vi "DPO_7K_Set_Channel_Bandwidth.vi"(8 "Error In":errorcluster, 9 "Bandwidth":u16(ring) items=["500 MHz", "1 GHz", "2 GHz", "3 GHz", "4 GHz", "5 GHz", "6 GHz", "7 GHz", "8 GHz", "9 GHz", "10 GHz", "11 GHz", "12 GHz", "13 GHz", "14 GHz", "15 GHz", "16 GHz", "17 GHz", "18 GHz", "19 GHz", "20 GHz", "21 GHz", "22 GHz", "23 GHz", "24 GHz", "25 GHz", "26 GHz", "27 GHz", "28 GHz", "29 GHz", "30 GHz", "31 GHz", "32 GHz", "33 GHz", "33 GHz HW (Tek)", "34 GHz (ATI)", "35 GHz (ATI)", "36 GHz (ATI)", "38 GHz (ATI)", "40 GHz (ATI)", "45 GHz (ATI)", "50 GHz (ATI)"], 10 "Channel":u16(ring) items=["Channel 1", "Channel 2", "Channel 3", "Channel 4", "Math 1", "Math 2", "Math 3", "Math 4", "Reference 1", "Reference 2", "Reference 3", "Reference 4"], 11 "VISA resource name in":refnum<visa-resource-name>) -> (0 "Error Out":errorcluster, 3 "VISA resource name out":refnum<visa-resource-name>)   [LabVIEW 2020]
uses:
  subVI/Return_To_Interface.ctl
  subVI/Set_Configuration.ctl
panel:
  in  "Set":T1
  in  "Return to Interface":T2
  # "SET CHANNEL BANDWIDTH"
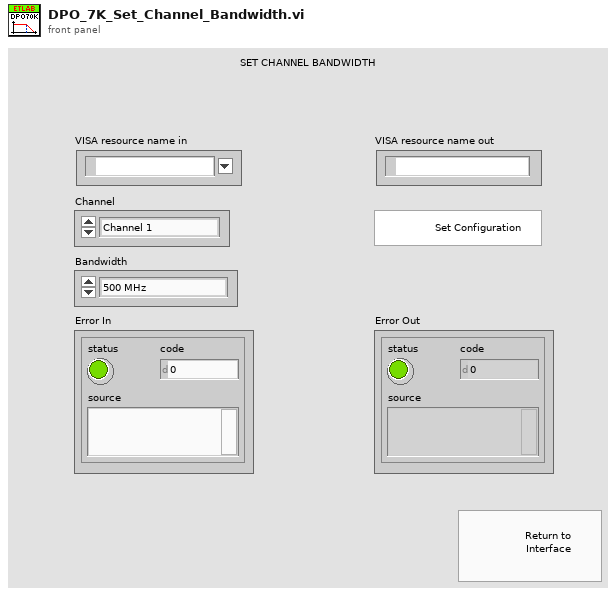
[diagram p1: front panel]
types:
  T1 = typedef "Set_Configuration.ctl" = bool
  T2 = typedef "Return_To_Interface.ctl" = bool
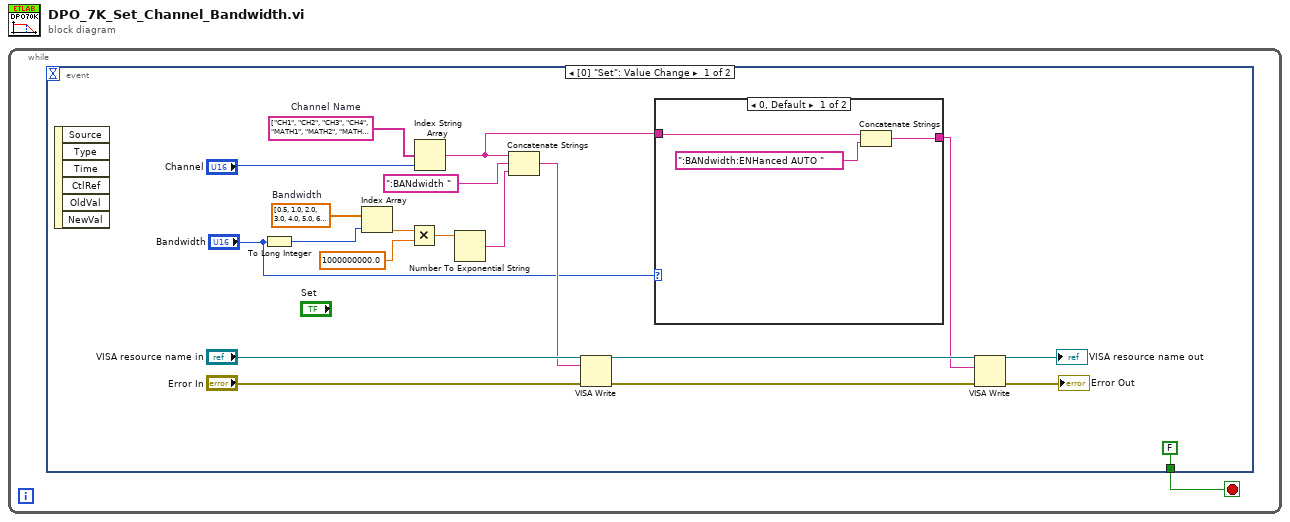
[diagram p0: block diagram]
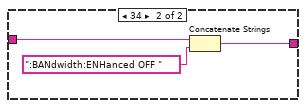
[diagram p2: hidden frame]
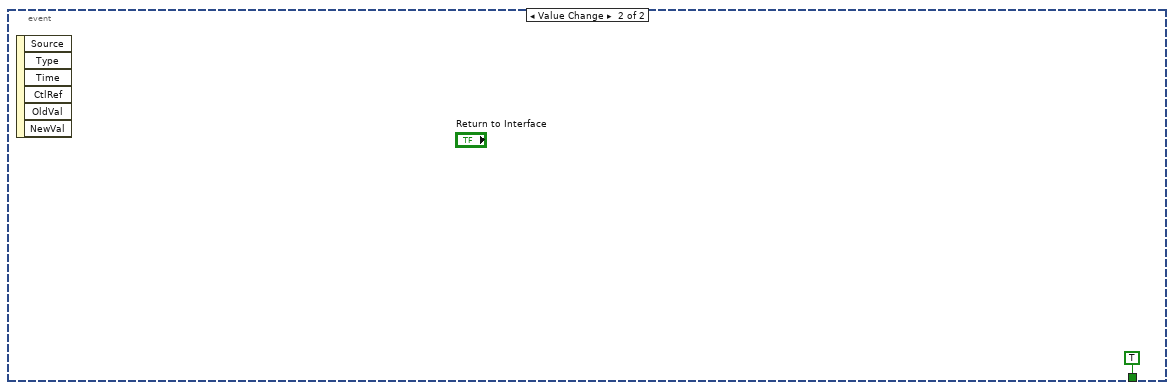
[diagram p3: hidden frame]
diagram:
  n1 = while {
    stop <- w1 stop-if-true
    n2 = event shown="[0] \"Set\": Value Change" {
      selector: _ -> [_ _]
      dyn-events: _ -> [_ _]
      timeout: _ -> [_ _]
      tunnel: [FALSE TRUE] -> w1
      event Value Change {
        w13 = dbl[] [0.5, 1.0, 2.0, 3.0, 4.0, 5.0, 6.0, 7.0, 8.0, 9.0, 10.0, 11.0, 12.0, 13.0, 14.0, 15.0, 16.0, 17.0, 18.0, 19.0, 20.0, 21.0, 22.0, 23.0, 24.0, 25.0, 26.0, 27.0, 28.0, 29.0, 30.0, 31.0, 32.0, 33.0, 33.0, 34.0, 35.0, 36.0, 38.0, 40.0, 45.0, 50.0]  # Bandwidth
        w18 = string[] ["CH1", "CH2", "CH3", "CH4", "MATH1", "MATH2", "MATH3", "MATH4", "REF1", "REF2", "REF3", "REF4"]  # Channel Name
        n3 = event-data() -> ()  [unwired: 1 in, 6 out]
        n4 = To Long Integer(number="Bandwidth") -> (32bit integer=w12:i32)
        n5 = Index Array(array=w13, index=w12) -> (element=w11:dbl)
        n6 = Multiply(x=w11, y=1000000000.0) -> (x*y=w9:dbl)
        n7 = Index String Array(1:"Channel", 2:w18) -> (0:w5:string)  [unwired: 1 in]
        n8 = Number To Exponential String(number=w9) -> (E-format string=w14:string)  [unwired: 3 in]
        n9 = Concatenate Strings(w5, ":BANdwidth ", w14) -> (w15:string)
        n10 = VISA Write(VISA resource name="VISA resource name in", write buffer=w15, error in (no error)="Error In") -> (VISA resource name out=w4:refnum<visa-resource-name>, error out=w3:errorcluster)  [unwired: 1 out]
        n11 = case shown="0, Default" "Bandwidth" {
          tunnel: w5 -> [w23 w27]
          tunnel: [w22 w25] -> w2
          frame 0, Default {
            n12 = Concatenate Strings(w23, ":BANdwidth:ENHanced AUTO ") -> (w22:string)
          }
          frame 34 {
            n13 = Concatenate Strings(w27, ":BANdwidth:ENHanced OFF ") -> (w25:string)
          }
        }
        n14 = VISA Write(VISA resource name=w4, write buffer=w2, error in (no error)=w3) -> (VISA resource name out=→"VISA resource name out":refnum<visa-resource-name>, error out=→"Error Out":errorcluster)  [unwired: 1 out]
      }
      event Value Change {
        n15 = event-data() -> ()  [unwired: 1 in, 6 out]
      }
    }
  }
